vi "Disconnect.vi"(8 "error in (no error)":errorcluster, 10 "Params":variant, 11 "Switching in":refnum<class "PIPXI40 GP Switch.lvclass">) -> (0 "error out":errorcluster, 3 "Switching out":refnum<class "PIPXI40 GP Switch.lvclass">)   [LabVIEW 2020, in "PIPXI40.lvlib" / "PIPXI40 GP Switch.lvclass"]
uses:
  PIPXI40 GP Switch.lvclass
  D:/WSGitHub/RTFWK/Realization/PIPXI40 Base/PIPXI40 Base.lvclass
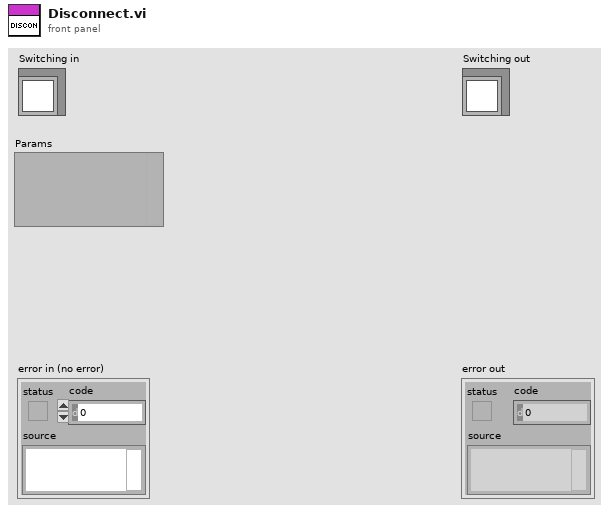
[diagram p1: front panel]
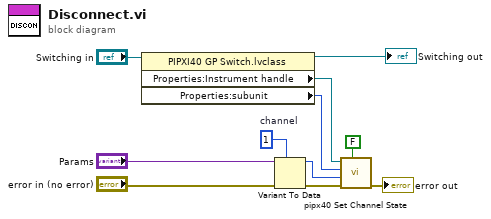
[diagram p0: block diagram]
diagram:
  w6 = u32 1  # channel
  n1 = property class="PIPXI40 GP Switch.lvclass"(reference="Switching in") -> (reference out=→"Switching out":refnum<class "PIPXI40 GP Switch.lvclass">, "Properties:Instrument handle"=w3:refnum<visa-resource-name>, "Properties:subunit"=w1:u32)  [unwired: 1 in, 1 out]
  n2 = Variant To Data(error in="error in (no error)", type=w6, Variant="Params") -> (data=w2:u32, error out=w11:errorcluster)
  n3 = call <instrlib>:"pipx40 Set Channel State.vi"("action"=FALSE, "error in (no error)"=w11, "channel number"=w2, "subunit number"=w1, "instrument handle"=w3) -> ("error out"=→"error out":errorcluster)  [unwired: 5 in, 1 out]
